vi "SDCP SMF Receiver andTransmitter - FTOR.vi"(4 "error in (no error)":errorcluster, 5 "Number of requested frames":refnum<vi>, 6 "Request frames":refnum<vi>, 7 "FTOR FIDs":refnum<vi>) -> (0 "error out":errorcluster)   [LabVIEW 2020]
uses:
  Typedefs/SDCP SMF logger - SMF with timestamp.ctl
panel:
  out "Received frames":u8[][](array[numeric])
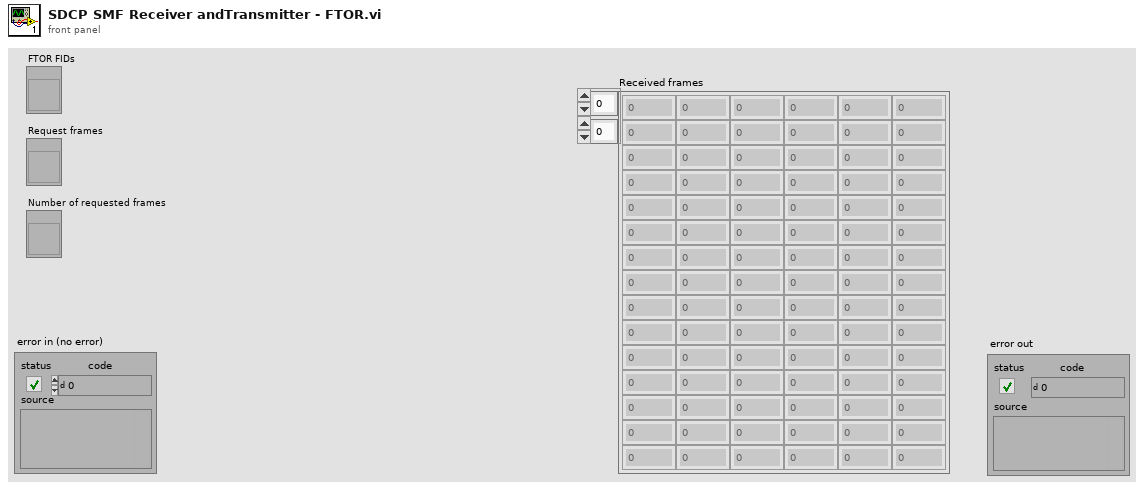
[diagram p1: front panel]
types:
  T1 = typedef "SDCP SMF Receiver and Transmitter - Notifier and Queues.ctl" = cluster{"Trace Queue":refnum<queue>, "Tx - Log Table Queue":refnum<queue>, "Tx - User Queue":refnum<queue>, "Rx - Log Table Queue":refnum<queue>, "Rx - User Queue":refnum<queue>, "Log status Notifier":refnum<notifier>, "Plot Queue":refnum<queue>}
  T2 = typedef "SDCP SMF logger - SMF with timestamp.ctl" = cluster{"Bytes":u8[], "Checksum":bool, "Time (ms)":u32, "Tx/Rx":string}
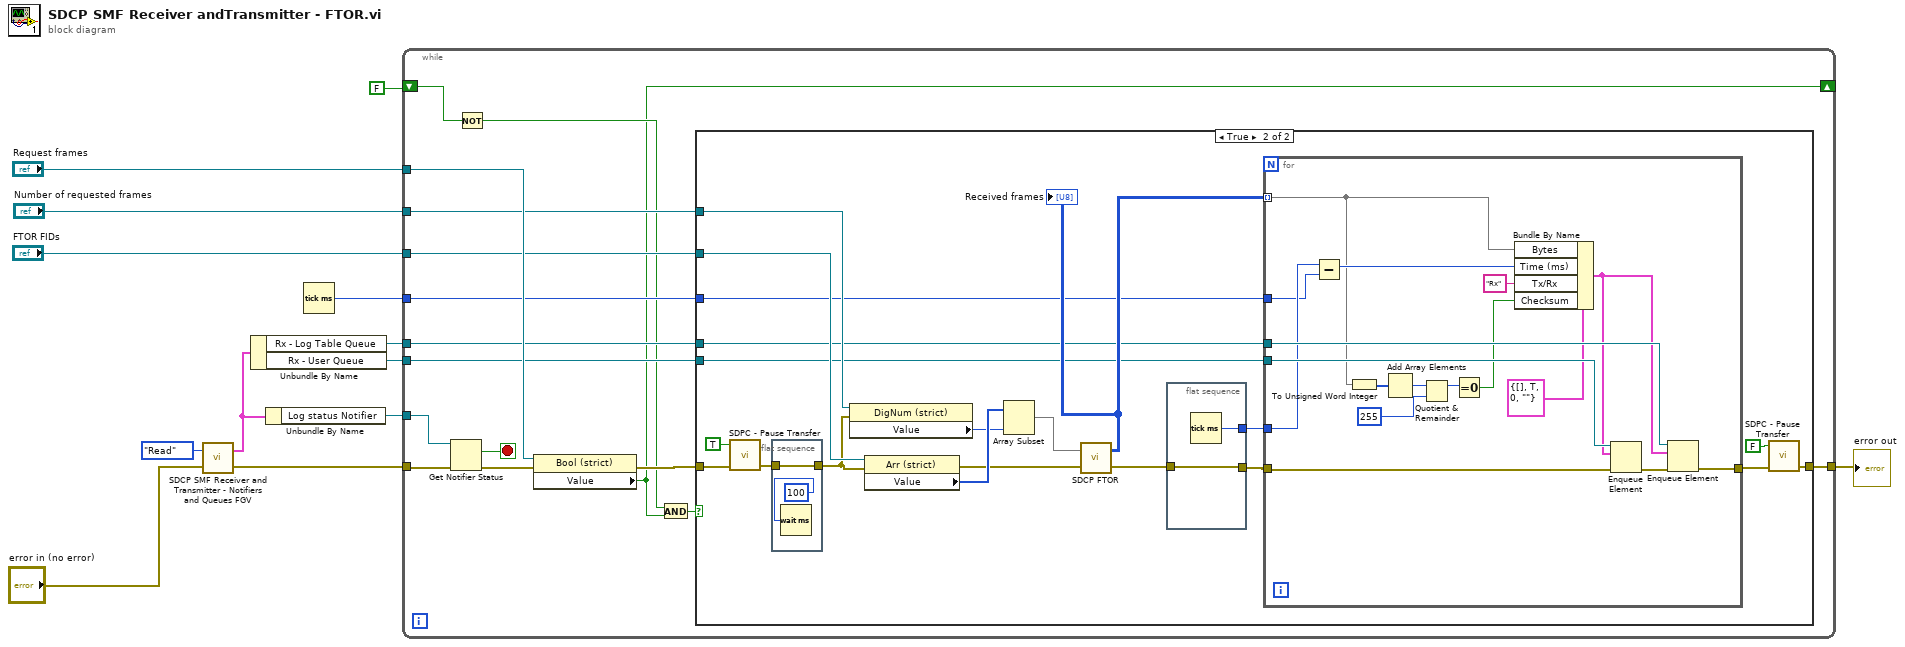
[diagram p0: block diagram]
diagram:
  n1 = call "SDCP SMF Receiver and Transmitter - Notifiers and Queues FGV.vi"("error in (no error)"="error in (no error)", "Command"=enum16{"Initialize", "Read", "Deinitialize"}."Read") -> ("error out"=w11:errorcluster, "Output"=w5:T1)
  n2 = Unbundle By Name(w5) -> ("Rx - Log Table Queue"=w4:refnum<queue>, "Rx - User Queue"=w3:refnum<queue>)
  n3 = Unbundle By Name(w5) -> ("Log status Notifier"=w10:refnum<notifier>)
  n4 = Tick Count (ms)() -> (millisecond timer value=w2:u32)
  n5 = while {
    tunnel: w11 -> [w29]
    tunnel: w10 -> [w28]
    tunnel: "Request frames" -> [w25]
    tunnel: [w23] -> w8
    tunnel: "FTOR FIDs" -> [w22]
    tunnel: "Number of requested frames" -> [w21]
    tunnel: w4 -> [w20]
    tunnel: w3 -> [w19]
    tunnel: w2 -> [w18]
    shift-right: [w14] -> _
    shift-left: FALSE -> [w17]
    stop <- w27 stop-if-true
    n6 = Get Notifier Status(notifier=w28, error in (no error)=w29) -> (current notification=w27:bool, error out=w26:errorcluster)  [unwired: 3 out]
    n7 = Not(x=w17) -> (.not. x?=w16:bool)
    n8 = property class="Bool (strict)"(reference=w25, error in=w26) -> (error out=w24:errorcluster, "Value"=w14:bool)  [unwired: 1 out]
    n9 = And(x=w16, y=w14) -> (x .and. y?=w15:bool)
    n10 = case shown="True" w15 {
      tunnel: w24 -> [w30 w50]
      tunnel: [w30 w35] -> w23
      tunnel: w22 -> [_ w48]
      tunnel: w21 -> [_ w47]
      tunnel: w20 -> [_ w39]
      tunnel: w19 -> [_ w38]
      tunnel: w18 -> [_ w37]
      frame False {
      }
      frame True {
        n11 = call "SDPC - Pause Transfer.vi"("error in (no error)"=w50, "Pause transfer"=TRUE) -> ("error out"=w42:errorcluster)  [unwired: 2 in, 1 out]
        n12 = flat-sequence {
          tunnel: w42 -> [w71]
          tunnel: [w71] -> w41
          frame #0 {
            n13 = Wait (ms)(milliseconds to wait=u32 100) -> ()  [unwired: 1 out]
          }
        }
        n14 = property class="DigNum (strict)"(reference=w47, error in=w41) -> ("Value"=w45:u8)  [unwired: 2 out]
        n15 = property class="Arr (strict)"(reference=w48, error in=w41) -> (error out=w44:errorcluster, "Value"=w46:u8[])  [unwired: 1 out]
        n16 = Array Subset(array=w46, length=w45) -> (w43:u8[])  [unwired: 1 in]
        n17 = call "SDCP FTOR.vi"("error in (no error)"=w44, "FID"=w43) -> ("error out"=w33:errorcluster, "Received frames"=w40:u8[][])
        "Received frames" <- w40
        n18 = flat-sequence {
          tunnel: w33 -> [w52]
          tunnel: [w52] -> w32
          tunnel: [w51] -> w31
          frame #0 {
            n19 = Tick Count (ms)() -> (millisecond timer value=w51:u32)
          }
        }
        n20 = for {
          tunnel: w32 -> [w68]
          tunnel: w40 -> [w58] mode=indexing
          tunnel: w39 -> [w65]
          tunnel: w38 -> [w66]
          tunnel: w37 -> [w62]
          tunnel: [w69] -> w34
          tunnel: w31 -> [w63]
          n21 = Subtract(x=w63, y=w62) -> (x-y=w61:u32)
          n22 = To Unsigned Word Integer(number=w58) -> (unsigned 16bit integer=w57:u16[])
          n23 = Add Array Elements(numeric array=w57) -> (sum=w56:u16)
          n24 = Quotient & Remainder(x=w56, y=u16 255) -> (x-y*floor(x/y)=w54:u16)  [unwired: 1 out]
          n25 = Equal To 0?(x=w54) -> (x = 0?=w53:bool)
          n26 = Bundle By Name(cluster=T2 {"Bytes"=[], "Checksum"=TRUE, "Time (ms)"=0, "Tx/Rx"=""} ("element"), "Bytes"=w58, "Time (ms)"=w61, "Tx/Rx"="Rx", "Checksum"=w53) -> (w59:T2)
          n27 = Enqueue Element(queue=w66, element=w59, error in (no error)=w68) -> (error out=w67:errorcluster)  [unwired: 1 in, 2 out]
          n28 = Enqueue Element(queue=w65, element=w59, error in (no error)=w67) -> (error out=w69:errorcluster)  [unwired: 1 in, 2 out]
        }
        n29 = call "SDPC - Pause Transfer.vi"("error in (no error)"=w34, "Pause transfer"=FALSE) -> ("error out"=w35:errorcluster)  [unwired: 2 in, 1 out]
      }
    }
  }
  "error out" <- w8
